vi "Power On.vi"(8 "error in (no error)":errorcluster, 11 "Dual Fan in":refnum<class "Dual Fan.lvclass">) -> (0 "error out":errorcluster, 3 "Dual Fan out":refnum<class "Dual Fan.lvclass">)   [LabVIEW 2012, in "Dual Fan.lvlib" / "Dual Fan.lvclass"]
uses:
  Dual Fan.lvclass
  Dual Fan.lvclass/Dual Fan.ctl
  Simulation/Simulation Data_Global.vi
  Simulation/Simulation.lvlib
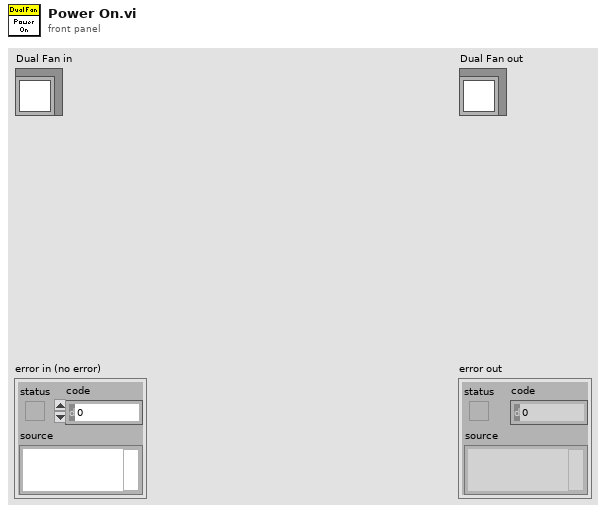
[diagram p1: front panel]
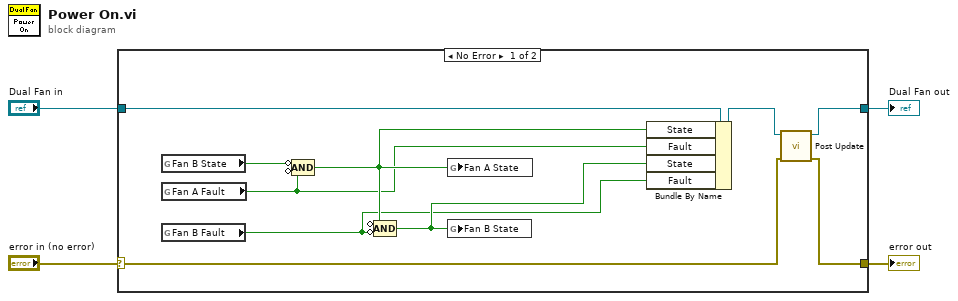
[diagram p0: block diagram]
diagram:
  n1 = case shown="No Error" "error in (no error)" {
    selector: "error in (no error)" -> [w6 w16]
    tunnel: [w5 w16] -> w3
    tunnel: [w7 w15] -> w1
    tunnel: "Dual Fan in" -> [w14 w15]
    frame No Error {
      n2 = global read "Simulation Data_Global.vi" "Fan B State"() -> (w9:bool)
      n3 = global read "Simulation Data_Global.vi" "Fan A Fault"() -> (w11:bool)
      n4 = global read "Simulation Data_Global.vi" "Fan B Fault"() -> (w10:bool)
      n5 = Compound Arithmetic op=AND(invert w9, invert w11) -> (w12:bool)
      n6 = Compound Arithmetic op=AND(invert w12, invert w10) -> (w13:bool)
      n7 = global write "Simulation Data_Global.vi" "Fan A State"(w12) -> ()
      n8 = global write "Simulation Data_Global.vi" "Fan B State"(w13) -> ()
      n9 = Bundle By Name(cluster=w14, "State"=w12, "Fault"=w11, "State"=w13, "Fault"=w10) -> (w8:refnum<class "Dual Fan.lvclass">)
      n10 = call "Post Update.vi"("error in (no error)"=w6, "Dual Fan in"=w8) -> ("error out"=w5:errorcluster, "Dual Fan out"=w7:refnum<class "Dual Fan.lvclass">)  [unwired: 8 in]
    }
    frame Error {
    }
  }
  "error out" <- w3
  "Dual Fan out" <- w1
